vi "Turner_PCO_CamExample.vi"() -> ()   [LabVIEW 2020]
uses:
  <userlib>/PCO LabVIEW 5.0.0/pco.camera/Controls/binning.ctl
  <userlib>/PCO LabVIEW 5.0.0/pco.camera/Camera.lvclass
  <vilib>/DAQmx/create/channels.llb/DAQmx Create Channel (CO-Pulse Generation-Frequency).vi
  <vilib>/DAQmx/configure/timing.llb/DAQmx Timing (Implicit).vi
panel:
  in  "roi":cluster{"x0":u64, "y0":u64, "x1":u64, "y1":u64}={"x0"=1, "y0"=1, "x1"=640, "y1"=540}
  in  "binning":T1={"vert"=4, "horz"=4}
  in  "TriggerMode":T2(ring)=enum."external exposure start"
  in  "Exposure Time [s]":dbl=0.0005 min=0.0005 max=2.0 step=0.001
  out "Recording On":bool=TRUE
  out "Filename":string="230228_13_26_57"
  in  "Time (min)":dbl(knob)=0.1 min=0.1 max=20.0 step=0.1 scale=0.0..20.0 scale format="%#_2g"
  in  "File Path":path=path "C:/Users/klt8/Documents/PCO Camera Tests" caption="Temporary Path for Streamed Data"
  in  "Sampling Rates":T3={"CBV Cam Fs"=30, "Whisk Cam Fs"=150, "Web Cam Fs"=30, "Pupil Cam Fs"=30}
  out "Image":T4(plugin-control)
  out "Recorded Images":u32=180
  # "Turner PCO Example"
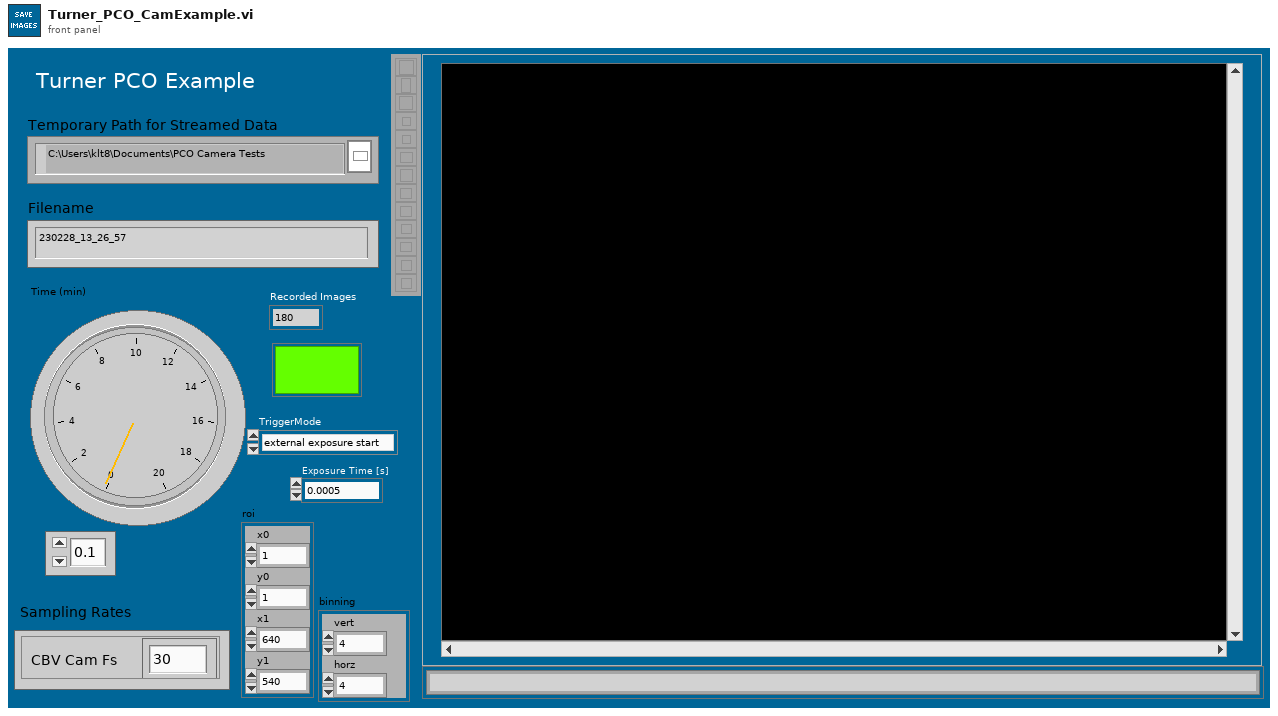
[diagram p1: front panel]
types:
  T1 = typedef "Camera.lvclass/binning.ctl" = cluster{"vert":u16, "horz":u16}
  T2 = enum16{"auto sequence", "software trigger", "external exposure start", "external exposure control"}
  T3 = cluster{"CBV Cam Fs":u16, "Whisk Cam Fs":u16, "Web Cam Fs":u16, "Pupil Cam Fs":u16}
  T4 = typedef "IMAQ Image.ctl" = refnum<image>
  T5 = enum16{"sequence", "sequence non blocking", "ring buffer", "fifo", "sequence_dpcore", "sequence_non_blocking_dpcore", "ring_buffer_dpcore", "fifo_dpcore", "tif", "multitif", "pcoraw", "b16", "dicom", "multidicom"}
  T6 = enum16{"Undefined", "Mono8", "Mono16", "BGRA8", "RGBA8", "BGRA16", "RGBA16", "CompressedMono8"}
  T7 = typedef "Image Type" = u32
  T8 = cluster{"exposure_time_s":dbl, "delay_time_s":dbl, "roi":cluster{"x0":u64, "y0":u64, "x1":u64, "y1":u64}, "timestamp_mode":u16, "pixelrate":u32, "trigger_mode":u16, "acquire_mode":u16, "metadata_mode":u16, "noisefilter_mode":u16, "binning":T1}
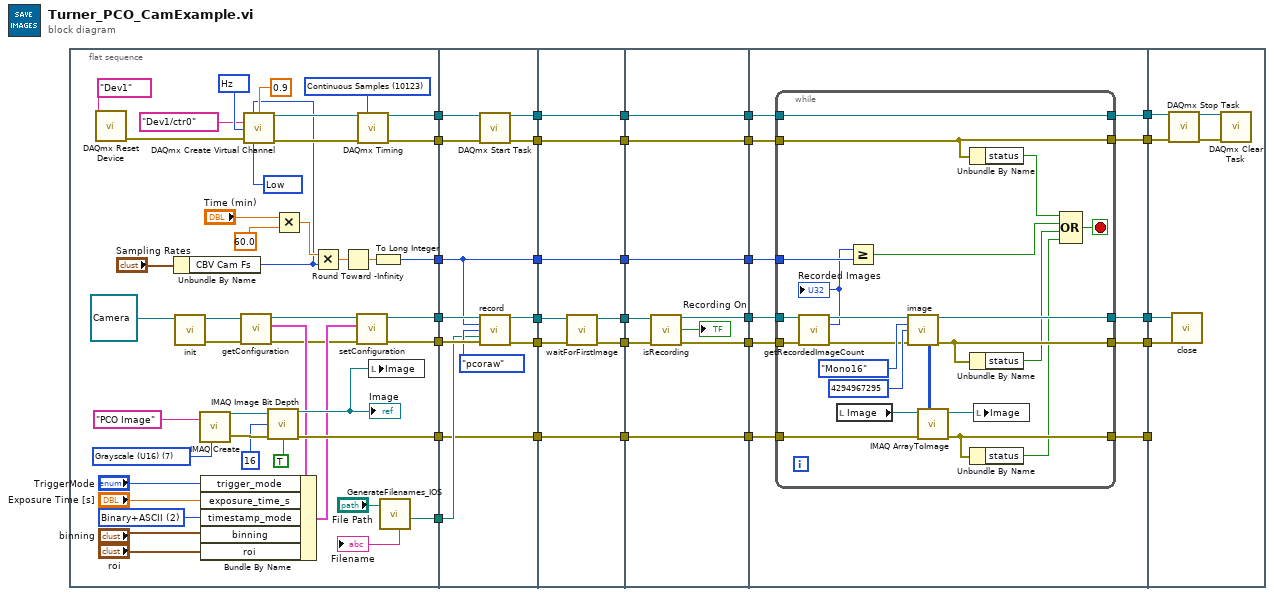
[diagram p0: block diagram]
diagram:
  n1 = flat-sequence {
    tunnel: [w35] -> w30
    tunnel: [w34] -> w29
    tunnel: [w57] -> w28
    tunnel: [w56] -> w27
    tunnel: [w55] -> w26
    tunnel: [w54] -> w25
    tunnel: [w45] -> w16
    tunnel: w30 -> [w86]
    tunnel: w29 -> [w85]
    tunnel: [w84] -> w14
    tunnel: [w83] -> w12
    tunnel: w28 -> [w76]
    tunnel: w27 -> [w81]
    tunnel: w26 -> [w80]
    tunnel: w25 -> [w79]
    tunnel: [w78] -> w10
    tunnel: [w77] -> w8
    tunnel: [w76] -> w6
    tunnel: [w75] -> w4
    tunnel: w16 -> [w75]
    tunnel: w14 -> [w90]
    tunnel: [w89] -> w13
    tunnel: w12 -> [w87]
    tunnel: [w88] -> w11
    tunnel: w10 -> [w94]
    tunnel: [w94] -> w9
    tunnel: w8 -> [w93]
    tunnel: [w93] -> w7
    tunnel: w6 -> [w92]
    tunnel: [w92] -> w5
    tunnel: w4 -> [w91]
    tunnel: [w91] -> w3
    tunnel: w13 -> [w98]
    tunnel: w11 -> [w99]
    tunnel: [w103] -> w24
    tunnel: w9 -> [w103]
    tunnel: [w102] -> w23
    tunnel: w7 -> [w102]
    tunnel: w5 -> [w101]
    tunnel: [w101] -> w18
    tunnel: [w100] -> w17
    tunnel: w3 -> [w100]
    tunnel: [w96] -> w2
    tunnel: [w95] -> w1
    tunnel: w24 -> [w111]
    tunnel: w23 -> [w110]
    tunnel: [w109] -> w22
    tunnel: [w114] -> w21
    tunnel: [w113] -> w20
    tunnel: [w112] -> w19
    tunnel: w18 -> [w108]
    tunnel: w17 -> [w107]
    tunnel: [w106] -> w15
    tunnel: w2 -> [w105]
    tunnel: w1 -> [w104]
    tunnel: w22 -> [w142]
    tunnel: w21 -> [w138]
    tunnel: w20 -> [w137]
    tunnel: w19 -> [w141]
    tunnel: w15 -> [_]
    frame #0 {
      w42 = u16 2 items=["OFF", "Binary", "Binary+ASCII", "ASCII"] ("wTimeStampMode")
      w52 = T7 7 items=["Grayscale (U8)", "Grayscale (I16)", "Grayscale (SGL)", "Complex (CSG)", "RGB (U32)", "HSL (U32)", "RGB (U64)", "Grayscale (U16)"] ("Image Type")
      w68 = 10123 items=["Finite Samples"=10178, "Continuous Samples"=10123, "Hardware Timed Single Point"=12522] ("sample mode")
      w71 = 10373 items=["Hz"=10373] ("units")
      w72 = 10214 items=["High"=10192, "Low"=10214] ("idle state")
      n2 = call <vilib>:"DAQmx Reset Device.vi"("device in"=tag "Dev1" ("NI Board")) -> ("error out"=w44:errorcluster)  [unwired: 14 in]
      n3 = Unbundle By Name("Sampling Rates") -> ("CBV Cam Fs"=w46:u16)
      n4 = call-dynamic "init.vi"("Camera in"=refnum<class "Camera.lvclass"> refnum ("PCOCamera in")) -> ("Camera out"=w37:refnum<class "Camera.lvclass">, "error out"=w36:errorcluster)  [unwired: 8 in]
      n5 = call "IMAQ Create"("Image Name"="PCO Image", "Image Type"=w52) -> ("New Image"=w51:T4, "error out"=w50:errorcluster)  [unwired: 3 in]
      n6 = call-dynamic "getConfiguration.vi"("error in (no error)"=w36, "Camera in"=w37) -> ("error out"=w33:errorcluster, "configuration"=w43:T8, "Camera out"=w39:refnum<class "Camera.lvclass">)  [unwired: 7 in]
      n7 = Bundle By Name(cluster=w43, "trigger_mode"="TriggerMode", "exposure_time_s"="Exposure Time [s]", "timestamp_mode"=w42, "binning"="binning", "roi"="roi") -> (w38:T8)
      n8 = call-poly <vilib>:"DAQmx Create Virtual Channel.vi"("frequency"=w46, "duty cycle"=0.9, "counter"=tag "Dev1/ctr0" ("Trig Source"), "units"=w71, "error in"=w44, "idle state"=w72) -> ("task out"=w70:refnum<k21>, "error out"=w69:errorcluster)  [unwired: 8 in]
      n9 = call "IMAQ Image Bit Depth"("Image"=w51, "Bit Depth (0)"=u32 16, "error in (no error)"=w50, "Get/Set Bit Depth? (Set)"=TRUE) -> ("Image Out"=w53:T4, "error out"=w45:errorcluster)  [unwired: 9 in, 1 out]
      "Image" <- w53
      n10 = Multiply(x="Time (min)", y=60.0) -> (x*y=w60:dbl)
      n11 = Multiply(x=w60, y=w46) -> (x*y=w59:dbl)
      n12 = Round Toward -Infinity(1:w59) -> (0:w58:dbl)
      n13 = call-dynamic "setConfiguration.vi"("error in (no error)"=w33, "configuration"=w38, "Camera in"=w39) -> ("error out"=w34:errorcluster, "Camera out"=w35:refnum<class "Camera.lvclass">)  [unwired: 7 in]
      n14 = call-poly <vilib>:"DAQmx Timing.vi"("task/channels in"=w70, "sample mode"=w68, "error in"=w69) -> ("task out"=w55:refnum<k21>, "error out"=w54:errorcluster)  [unwired: 11 in]
      n15 = local write "Image"(w53) -> ()
      n16 = To Long Integer(number=w58) -> (32bit integer=w57:i32)
      n17 = call "GenerateFilenames_IOS.vi"("path"="File Path") -> ("Dalsa Path"=w56:path, "Analog file name"=→"Filename":string)  [unwired: 3 in, 6 out]
    }
    frame #1 {
      n18 = call <vilib>:"DAQmx Start Task.vi"("task/channels in"=w80, "error in"=w79) -> ("task out"=w77:refnum<k21>, "error out"=w78:errorcluster)  [unwired: 12 in]
      n19 = call-dynamic "record.vi"("Camera in"=w86, "num_images"=w76, "record_mode"=T5."pcoraw", "file_path"=w81, "error in (no error)"=w85) -> ("Camera out"=w84:refnum<class "Camera.lvclass">, "error out"=w83:errorcluster)  [unwired: 9 in]
    }
    frame #2 {
      n20 = call-dynamic "waitForFirstImage.vi"("error in (no error)"=w87, "Camera in"=w90) -> ("error out"=w88:errorcluster, "Camera out"=w89:refnum<class "Camera.lvclass">)  [unwired: 8 in]
    }
    frame #3 {
      n21 = call-dynamic "isRecording.vi"("Camera in"=w98, "error in (no error)"=w99) -> ("Camera out"=w96:refnum<class "Camera.lvclass">, "recording"=→"Recording On":bool, "error out"=w95:errorcluster)  [unwired: 11 in]
    }
    frame #4 {
      n22 = while {
        tunnel: [w128] -> w112
        tunnel: w111 -> [w128]
        tunnel: [w132] -> w109
        tunnel: w110 -> [w132]
        tunnel: w108 -> [w130]
        tunnel: [w136] -> w114
        tunnel: [w127] -> w113
        tunnel: w107 -> [w129]
        tunnel: [w125] -> w106
        tunnel: w105 -> [w122]
        tunnel: w104 -> [w121]
        stop <- w131 stop-if-true
        n23 = call-dynamic "getRecordedImageCount.vi"("Camera in"=w122, "error in (no error)"=w121) -> ("Camera out"=w120:refnum<class "Camera.lvclass">, "recorded_image_count"=w115:u32, "error out"=w119:errorcluster)  [unwired: 11 in]
        "Recorded Images" <- w115
        n24 = local read "Image"() -> (w135:T4)
        n25 = Greater Or Equal?(x=w115, y=w130) -> (x >= y?=w117:bool)
        n26 = call-dynamic "image.vi"("Camera in"=w120, "data_format"=T6."Mono16", "image_index"=u32 4294967295 ("dwImgIdx"), "error in (no error)"=w119) -> ("Camera out"=w136:refnum<class "Camera.lvclass">, "raw_image (U16)"=w134:u16[][], "error out"=w127:errorcluster)  [unwired: 4 in, 5 out]
        n27 = call "IMAQ ArrayToImage"("Image Pixels (U16)"=w134, "error in (no error)"=w129, "Image"=w135) -> ("error out"=w125:errorcluster, "Image Out"=w118:T4)  [unwired: 7 in]
        n28 = Unbundle By Name(w128) -> ("status"=w116:bool)
        n29 = Unbundle By Name(w127) -> ("status"=w126:bool)
        n30 = Unbundle By Name(w125) -> ("status"=w124:bool)
        n31 = local write "Image"(w118) -> ()
        n32 = Compound Arithmetic op=OR(w116, w117, w126, w124) -> (w131:bool)
      }
    }
    frame #5 {
      n33 = call <vilib>:"DAQmx Stop Task.vi"("task/channels in"=w142, "error in"=w141) -> ("task out"=w140:refnum<k21>, "error out"=w139:errorcluster)  [unwired: 12 in]
      n34 = call-dynamic "close.vi"("error in (no error)"=w137, "Camera in"=w138) -> ()  [unwired: 9 in, 1 out]
      n35 = call <vilib>:"DAQmx Clear Task.vi"("task in"=w140, "error in"=w139) -> ()  [unwired: 13 in, 1 out]
    }
  }
